vi "TAT_Varient Creater.vi"(8 "error in (no error)":errorcluster) -> (0 "error out":errorcluster)   [LabVIEW 2017]
uses:
  <vilib>/Utility/config.llb/NI_LVConfig.lvlib
panel:
  in  "SINGLE VARIENT":T1
  in  "Delete Square":bool
  in  "EDIT & SAVE":bool
  out "Varient Details":string[][](table)
  in  "HOME":bool
  in  "UPDATE TABLE":bool
  # "Varient Creater"
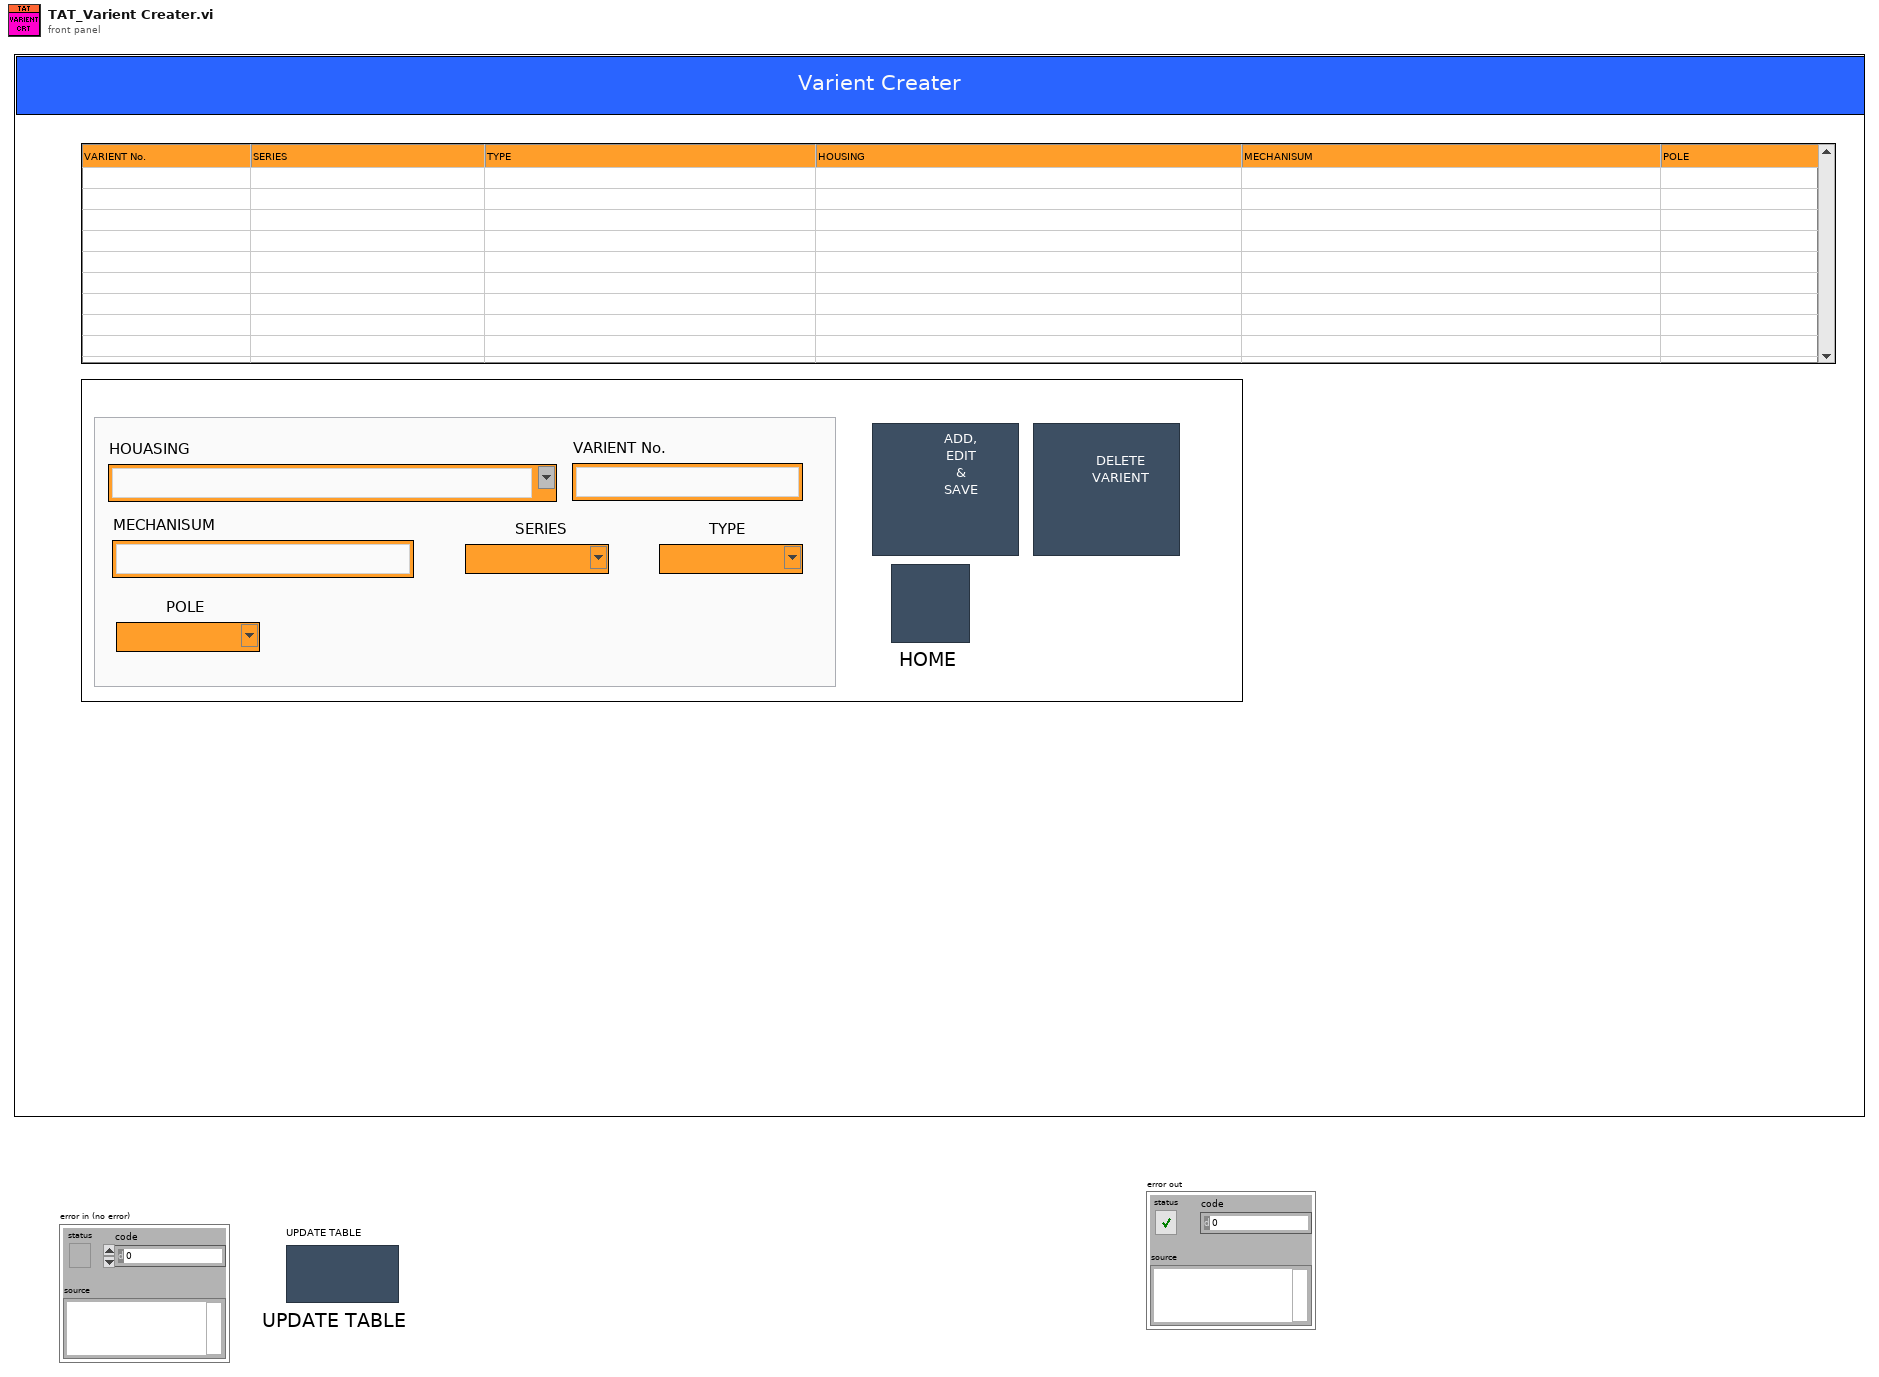
[diagram p1: front panel]
types:
  T1 = cluster{"HOUASING":string, "MECHANISUM":string, "VARIENT No.":string, "TYPE":string, "SERIES":string, "POLE":string}
  T2 = cluster{"RECIPE NO.":string, "CURVE":string, "HAMMER SPRING CAT NO":string, "SPRING FOR (N) MIN":dbl, "SPRING FOR (N) MAX":dbl}
  T3 = enum32{"invalid app kind", "Development System", "Run Time System", "Student Edition", "Embedded LabVIEW", "Evaluation", "Custom"}
  T4 = typedef "NI_LVConfig.lvlib/Config Data RefNum.ctl" = refnum<k1>
  T5 = typedef "LVComboBoxStrsAndValuesArrayTypeDef.ctl" = cluster{"String":string, "Value":string}[]
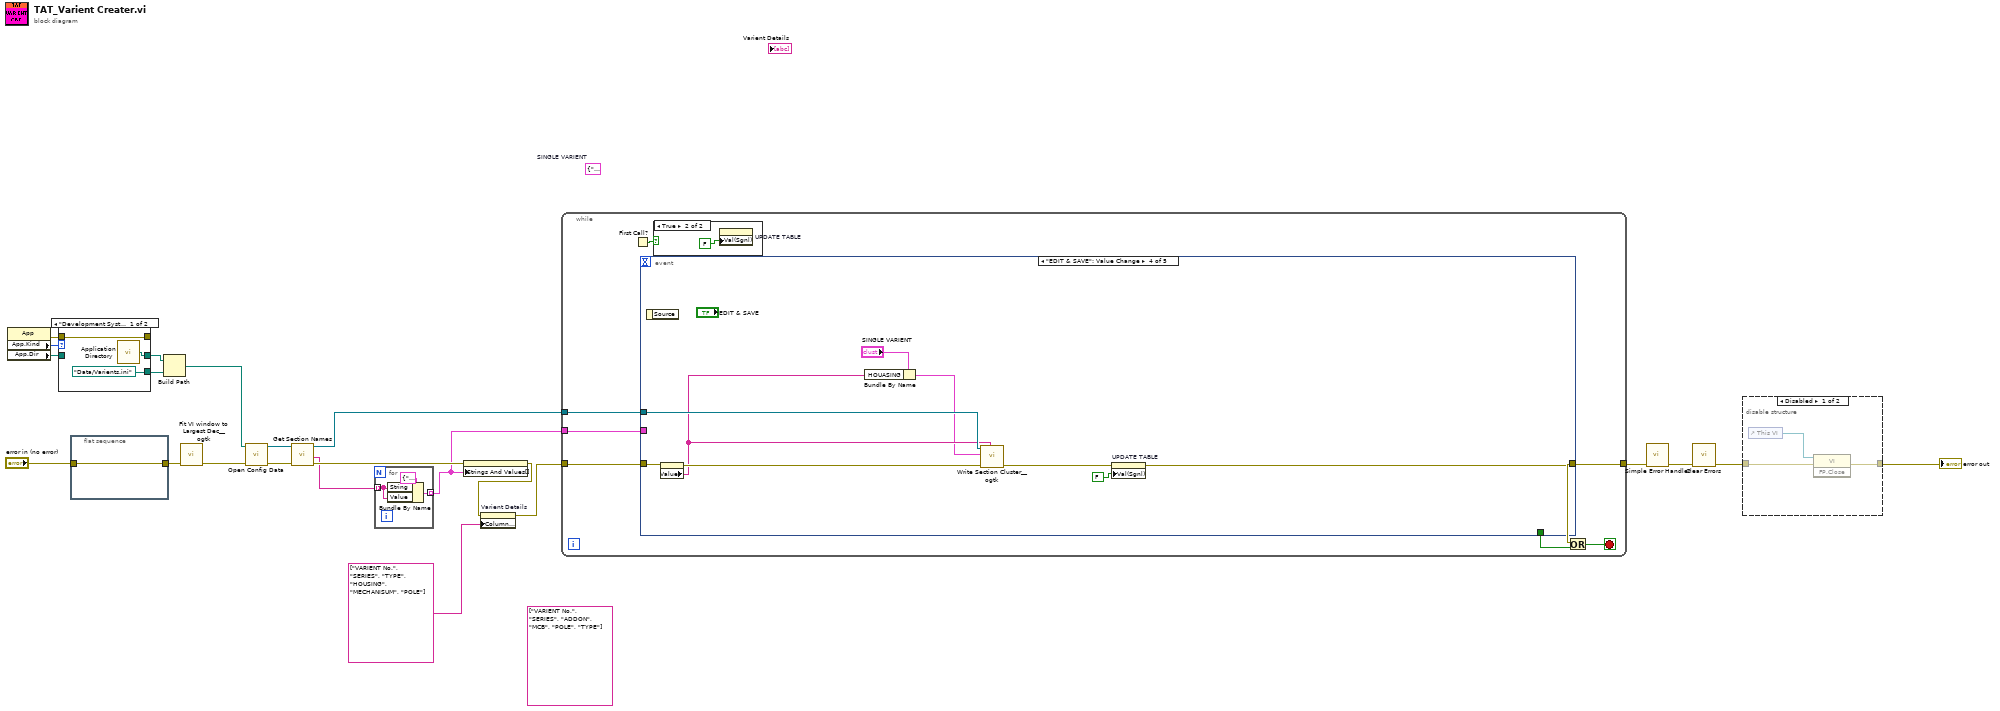
[diagram p0: block diagram]
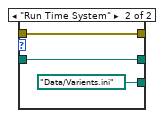
[diagram p2: hidden frame]
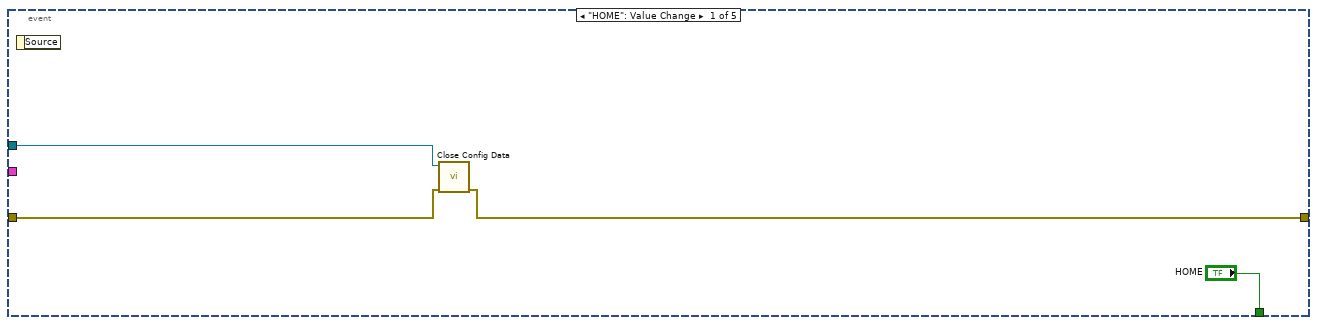
[diagram p5: hidden frame]
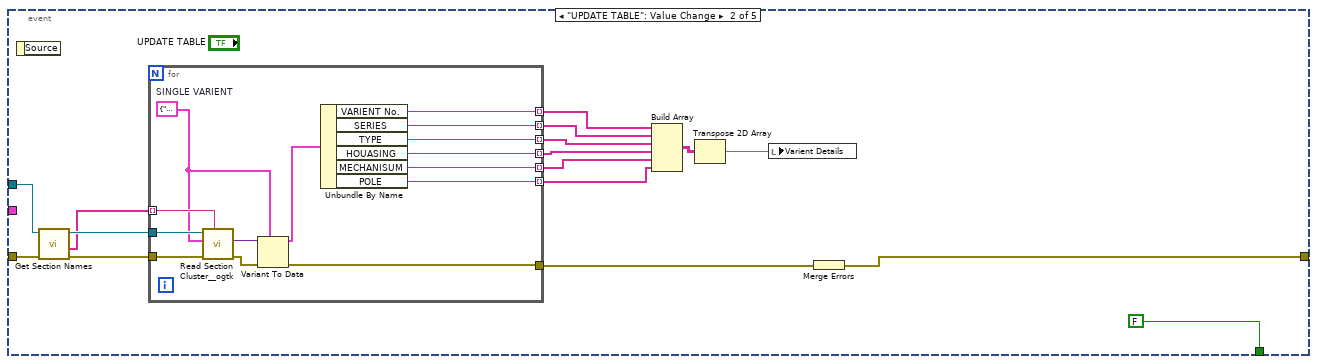
[diagram p6: hidden frame]
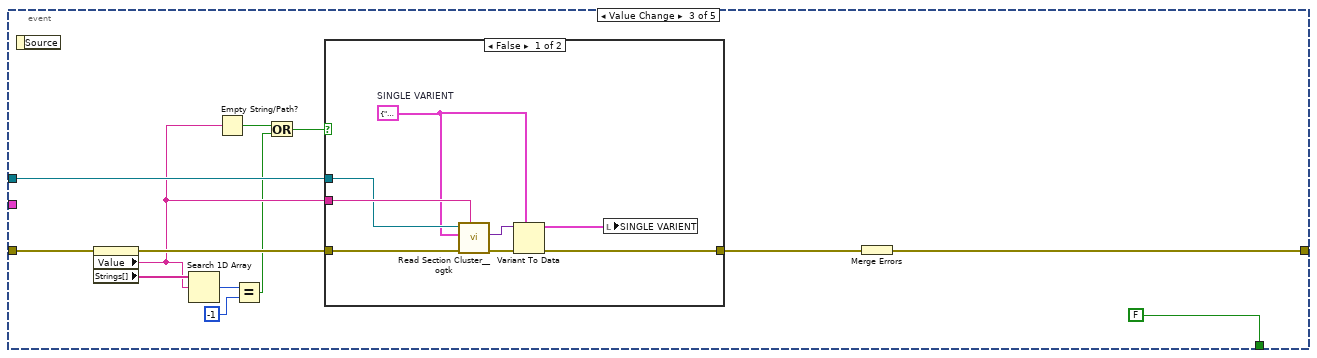
[diagram p7: hidden frame]
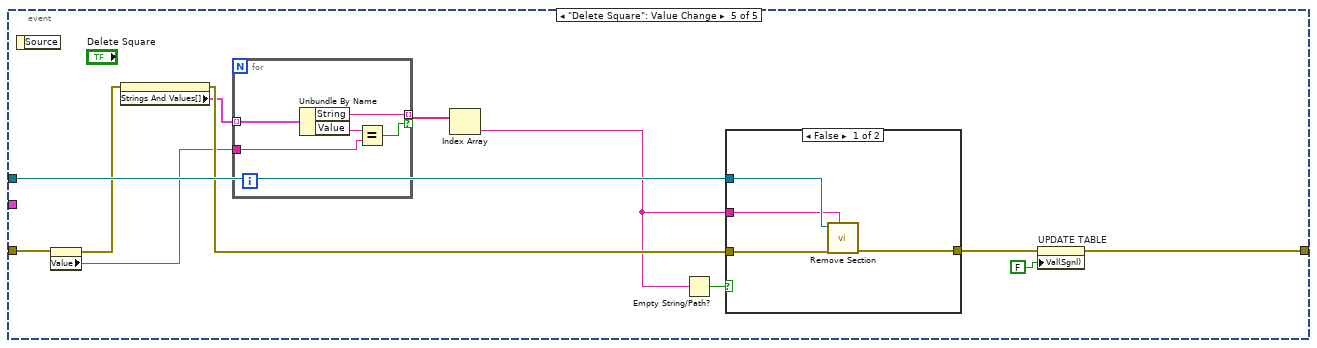
[diagram p9: hidden frame]
diagram:
  (unwired) string[] ["VARIENT No.", "SERIES", "ADDON", "MCB", "POLE", "TYPE"] ("Column Header Strings[]")
  (unwired) T2 {"RECIPE NO."="", "CURVE"="C", "HAMMER SPRING CAT NO"="XB02306", "SPRING FOR (N) MIN"=14.96, "SPRING FOR (N) MAX"=14.96}  # SINGLE VARIENT
  n1 = property class="App"() -> (error out=w8:errorcluster, "App.Kind"=w4:T3, "App.Dir"=w7:path)  [unwired: 2 in, 1 out]
  n2 = case shown="\"Development System\", Default" w4 {
    tunnel: [w25 w28] -> _
    tunnel: w8 -> [w25 w28]
    tunnel: w7 -> [_ w26]
    tunnel: [path "Data/Varients.ini" path "Data/Varients.ini"] -> w6
    tunnel: [w23 w26] -> w5
    frame "Development System", Default {
      n3 = call <vilib>:"Application Directory.vi"() -> ("Application Directory"=w23:path)
    }
    frame "Run Time System" {
    }
  }
  n4 = flat-sequence {
    tunnel: [w29] -> w10
    tunnel: "error in (no error)" -> [w29]
    frame #0 {
    }
  }
  n5 = Build Path(base path=w5, name or relative path=w6) -> (appended path=w3:path)
  n6 = call <userlib>:"Fit VI window to Largest Dec__ogtk.vi"("error in (no error)"=w10) -> ("error out"=w9:errorcluster)  [unwired: 5 in, 1 out]
  n7 = call <vilib>:"Open Config Data.vi"("error in (no error)"=w9, "configuration file path"=w3) -> ("error out"=w17:errorcluster, "refnum"=w18:T4)  [unwired: 7 in, 1 out]
  n8 = call <vilib>:"Get Section Names.vi"("error in (no error)"=w17, "refnum"=w18) -> ("error out"=w16:errorcluster, "section names"=w2:string[], "refnum out"=w15:T4)  [unwired: 7 in]
  n9 = for {
    tunnel: w2 -> [w31] mode=indexing
    tunnel: [w30] -> w1 mode=indexing
    n10 = Bundle By Name(cluster=cluster{"String":string, "Value":string} {"String"="", "Value"=""}, "String"=w31, "Value"=w31) -> (w30:cluster{"String":string, "Value":string})
  }
  n11 = property on="HOUASING" class="CmbBox"(error in=w16, "Strings And Values[]"=w1) -> (error out=w14:errorcluster)  [unwired: 1 in, 1 out]
  n12 = property on="Varient Details" class="Tbl (strict)"(error in=w14, "Column Headers[]"=string[] ["VARIENT No.", "SERIES", "TYPE", "HOUSING", "MECHANISUM", "POLE"] ("Column Header Strings[]")) -> (error out=w13:errorcluster)  [unwired: 1 in, 1 out]
  n13 = while {
    tunnel: w13 -> [w38]
    tunnel: [w36] -> w19
    tunnel: w15 -> [w35]
    tunnel: w1 -> [w33]
    stop <- w37 stop-if-true
    n14 = First Call?() -> (First Call?: T/F=w34:bool)
    n15 = event shown="[3] \"EDIT & SAVE\": Value Change" {
      selector: _ -> [_ _ _ _ _]
      dyn-events: _ -> [_ _ _ _ _]
      timeout: _ -> [_ _ _ _ _]
      tunnel: ["HOME" FALSE ("stop") FALSE ("stop") _ _] -> w39
      tunnel: w38 -> [w43 w59 w84 w105 w116]
      tunnel: [w42 w54 w85 w101 w112] -> w36
      tunnel: w35 -> [w41 w58 w82 w104 w117]
      tunnel: w33 -> [_ _ _ _ _]
      event "HOME": Value Change {
        n16 = event-data() -> ()  [unwired: 1 in, 1 out]
        n17 = call <vilib>:"Close Config Data.vi"("error in (no error)"=w43, "refnum"=w41) -> ("error out"=w42:errorcluster)  [unwired: 8 in, 1 out]
      }
      event "UPDATE TABLE": Value Change {
        n18 = event-data() -> ()  [unwired: 1 in, 1 out]
        n19 = call <vilib>:"Get Section Names.vi"("error in (no error)"=w59, "refnum"=w58) -> ("error out"=w56:errorcluster, "section names"=w47:string[], "refnum out"=w57:T4)  [unwired: 7 in]
        n20 = for {
          tunnel: w47 -> [w72] mode=indexing
          tunnel: w57 -> [w74]
          tunnel: w56 -> [w73]
          tunnel: [w69] -> w55
          tunnel: [w64] -> w53 mode=indexing
          tunnel: [w67] -> w52 mode=indexing
          tunnel: [w66] -> w51 mode=indexing
          tunnel: [w65] -> w50 mode=indexing
          tunnel: [w63] -> w46 mode=indexing
          tunnel: [w61] -> w45 mode=indexing
          w62 = T1 {"HOUASING"="", "MECHANISUM"="", "VARIENT No."="", "TYPE"="", "SERIES"="", "POLE"="2"}  # SINGLE VARIENT
          n21 = call <userlib>:"Read Section Cluster__ogtk.vi"("section (optional)"=w72, "error in (no error)"=w73, "Section Formatted Cluster Type"=w62, "refnum"=w74) -> ("error out"=w70:errorcluster, "Section Formatted Cluster"=w71:variant)  [unwired: 3 in, 3 out]
          n22 = Variant To Data(error in=w70, type=w62, Variant=w71) -> (data=w68:T1, error out=w69:errorcluster)
          n23 = Unbundle By Name(w68) -> ("VARIENT No."=w63:string, "SERIES"=w64:string, "TYPE"=w67:string, "HOUASING"=w66:string, "MECHANISUM"=w65:string, "POLE"=w61:string)
        }
        n24 = Build Array(w46, w53, w52, w51, w50, w45) -> (w49:string[][])
        n25 = Transpose 2D Array(2D array=w49) -> (transposed array=w48:string[][])
        n26 = local write "Varient Details"(w48) -> ()
        n27 = Merge Errors(w55) -> (w54:errorcluster)
      }
      event "SINGLE VARIENT.HOUASING": Value Change {
        n28 = event-data() -> ()  [unwired: 1 in, 1 out]
        n29 = property on="HOUASING" class="CmbBox"(error in=w84) -> (error out=w83:errorcluster, "Value"=w80:string, "Strings[]"=w81:string[])  [unwired: 1 in, 1 out]
        n30 = Search 1D Array(1D array=w81, element=w80) -> (index of element=w79:i32)  [unwired: 1 in]
        n31 = Empty String/Path?(string/path=w80) -> (empty?=w76:bool)
        n32 = Equal?(x=w79, y=-1) -> (x = y?=w75:bool)
        n33 = Or(x=w76, y=w75) -> (x .or. y?=w77:bool)
        n34 = case shown="False" w77 {
          tunnel: [w95 w96] -> w86
          tunnel: w83 -> [w94 w96]
          tunnel: w80 -> [w93 _]
          tunnel: w82 -> [w92 _]
          frame False {
            w88 = T1 {"HOUASING"="", "MECHANISUM"="", "VARIENT No."="", "TYPE"="", "SERIES"="", "POLE"="2"}  # SINGLE VARIENT
            n35 = call <userlib>:"Read Section Cluster__ogtk.vi"("section (optional)"=w93, "error in (no error)"=w94, "Section Formatted Cluster Type"=w88, "refnum"=w92) -> ("error out"=w90:errorcluster, "Section Formatted Cluster"=w91:variant)  [unwired: 3 in, 3 out]
            n36 = Variant To Data(error in=w90, type=w88, Variant=w91) -> (data=w89:T1, error out=w95:errorcluster)
            n37 = local write "SINGLE VARIENT"(w89) -> ()
          }
          frame True {
          }
        }
        n38 = Merge Errors(w86) -> (w85:errorcluster)
      }
      event "EDIT & SAVE": Value Change {
        n39 = event-data() -> ()  [unwired: 1 in, 1 out]
        n40 = property on="HOUASING" class="CmbBox"(error in=w105) -> (error out=w100:errorcluster, "Value"=w99:string)  [unwired: 1 in, 1 out]
        n41 = Bundle By Name(cluster="SINGLE VARIENT", "HOUASING"=w99) -> (w97:T1)
        n42 = call <userlib>:"Write Section Cluster__ogtk.vi"("section (optional)"=w99, "error in (no error)"=w100, "Section Formatted Cluster"=w97, "refnum"=w104) -> ("error out"=w102:errorcluster)  [unwired: 6 in, 1 out]
        n43 = property on="UPDATE TABLE" class="Bool (strict)"(error in=w102, "Val(Sgnl)"=FALSE) -> (error out=w101:errorcluster)  [unwired: 1 in, 1 out]
      }
      event "Delete Square": Value Change {
        n44 = event-data() -> ()  [unwired: 1 in, 1 out]
        n45 = property on="HOUASING" class="CmbBox"(error in=w116) -> (error out=w111:errorcluster, "Value"=w107:string)  [unwired: 1 in, 1 out]
        n46 = property on="HOUASING" class="CmbBox"(error in=w111) -> (error out=w110:errorcluster, "Strings And Values[]"=w109:T5)  [unwired: 1 in, 1 out]
        n47 = for {
          tunnel: w109 -> [w122] mode=indexing
          tunnel: w107 -> [w120]
          tunnel: [w119] -> w108 mode=indexing if=w118
          n48 = Unbundle By Name(w122) -> ("String"=w119:string, "Value"=w121:string)
          n49 = Equal?(x=w121, y=w120) -> (x = y?=w118:bool)
        }
        n50 = Index Array(array=w108) -> (element=w106:string)  [unwired: 1 in]
        n51 = Empty String/Path?(string/path=w106) -> (empty?=w115:bool)
        n52 = case shown="False" w115 {
          tunnel: [w126 w127] -> w113
          tunnel: w117 -> [w125 _]
          tunnel: w110 -> [w124 w127]
          tunnel: w106 -> [w123 _]
          frame False {
            n53 = call <vilib>:"Remove Section.vi"("section"=w123, "error in (no error)"=w124, "refnum"=w125) -> ("error out"=w126:errorcluster)  [unwired: 6 in, 2 out]
          }
          frame True {
          }
        }
        n54 = property on="UPDATE TABLE" class="Bool (strict)"(error in=w113, "Val(Sgnl)"=FALSE) -> (error out=w112:errorcluster)  [unwired: 1 in, 1 out]
      }
    }
    n55 = case shown="True" w34 {
      frame False {
      }
      frame True {
        n56 = property on="UPDATE TABLE" class="Bool (strict)"("Val(Sgnl)"=FALSE) -> ()  [unwired: 2 in, 2 out]
      }
    }
    n57 = Or(x=w36, y=w39) -> (x .or. y?=w37:bool)
  }
  n58 = call <vilib>:"Simple Error Handler.vi"("error in (no error)"=w19) -> ("error out"=w22:errorcluster)  [unwired: 4 in, 4 out]
  n59 = call <vilib>:"Clear Errors.vi"("error in (no error)"=w22) -> ("error out"=w21:errorcluster)  [unwired: 5 in, 1 out]
  n60 = disable-structure shown="Disabled" {
    disable-tunnel: w21 -> [w130 w131]
    disable-tunnel: [w129 w131] -> w20
    frame Disabled {
      n61 = control-ref of="This VI"() -> (w128:refnum<vi>)
      n62 = invoke class="VI" method="FP.Close"(reference=w128, error in=w130) -> (error out=w129:errorcluster)  [unwired: 1 in, 2 out]
    }
    frame Enabled {
    }
  }
  "error out" <- w20
